vi "Initialize JSON Schema.vi"(8 "error in (no error)":errorcluster, 11 "Variant":variant) -> (0 "error out":errorcluster, 3 "JSON Schema out":string)   [LabVIEW 2019, in "JSON-Schema.lvlib"]
uses:
  JSON-Schema.lvlib
  <vilib>/JDP Science/JSONtext/JSONtext.lvlib
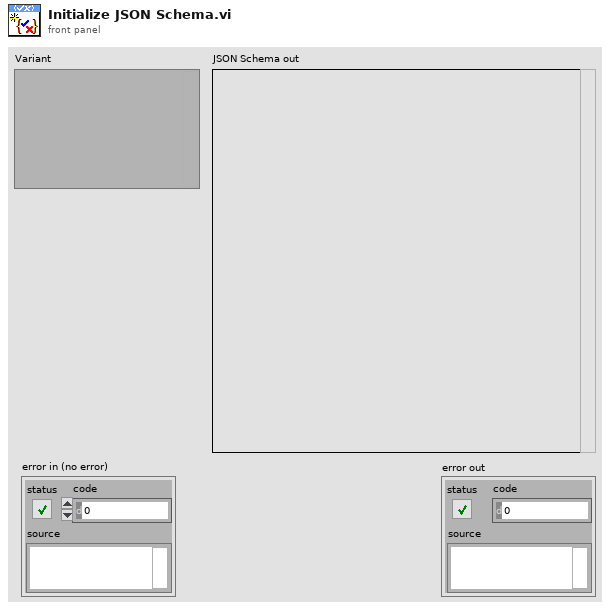
[diagram p1: front panel]
types:
  T1 = enum32{"Bad", "Idle", "Run top level", "Running"}
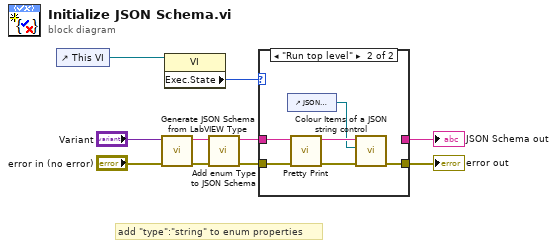
[diagram p0: block diagram]
diagram:
  # "add \"type\":\"string\" to enum properties"
  n1 = control-ref of="This VI"() -> (w6:refnum<vi>)
  n2 = call <vilib>:"Generate JSON Schema from LabVIEW Type.vi"("error in (no error)"="error in (no error)", "Variant"="Variant") -> ("error out"=w8:errorcluster, "JSON Schema"=w7:string)  [unwired: 8 in]
  n3 = property class="VI"(reference=w6) -> ("Exec.State"=w5:T1)  [unwired: 1 in, 2 out]
  n4 = call "Add enum Type to JSON Schema.vi"("error in (no error)"=w8, "JSON Schema in"=w7) -> ("error out"=w4:errorcluster, "JSON Schema out"=w3:string)  [unwired: 8 in]
  n5 = case shown="\"Run top level\"" w5 {
    tunnel: w3 -> [w11 w17]
    tunnel: w4 -> [w12 w16]
    tunnel: [w12 w14] -> w2
    tunnel: [w11 _] -> w1
    frame Default {
    }
    frame "Run top level" {
      n6 = control-ref of="JSON Schema out"() -> (w13:refnum<vi>)
      n7 = call <vilib>:"Pretty Print.vi"("error in (no error)"=w16, "JSON"=w17) -> ("error out"=w15:errorcluster, "<JSON>"=w18:string)  [unwired: 7 in, 1 out]
      n8 = call <vilib>:"Colour Items of a JSON string control.vi"("error in (no error)"=w15, "String Control"=w13, "JSON"=w18) -> ("error out"=w14:errorcluster)  [unwired: 8 in]
    }
  }
  "JSON Schema out" <- w1
  "error out" <- w2
